vi "LowestRow.vi"(9 "View":i32[](array[numeric]) caption="View (Team Index, -1: empty)", 10 "Team Index":i32) -> (1 "Is lowest":bool)   [LabVIEW 2015, in "AndrewF.lvclass"]
uses:
  AndrewF.lvclass
panel:
  # "NW\nN\nNE\nE\nSE\nS\nSW\nW"
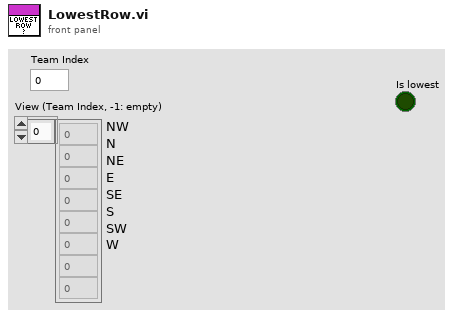
[diagram p1: front panel]
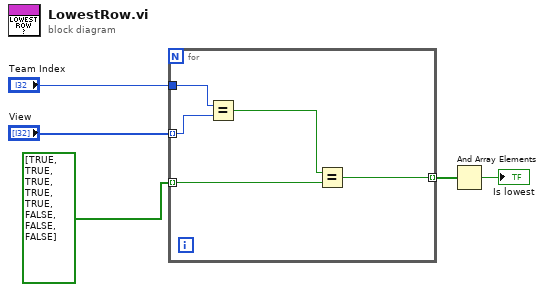
[diagram p0: block diagram]
diagram:
  n1 = for {
    tunnel: "Team Index" -> [w10]
    tunnel: "View" -> [w9] mode=indexing
    tunnel: bool[] [TRUE, TRUE, TRUE, TRUE, TRUE, FALSE, FALSE, FALSE] -> [w8] mode=indexing
    tunnel: [w6] -> w2 mode=indexing
    n2 = Equal?(x=w10, y=w9) -> (x = y?=w7:bool)
    n3 = Equal?(x=w7, y=w8) -> (x = y?=w6:bool)
  }
  n4 = And Array Elements(Boolean array=w2) -> (logical AND=→"Is lowest":bool)
